vi "ShiftLeft.vi"(11 "Array":i32[](array[numeric])=[0, 3, 2, 1]) -> (3 "Array 2":i32[](array[numeric])=[0, 3, 2, 1], 5 "tiles moved?":bool)   [LabVIEW 2021]
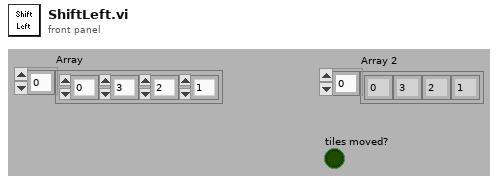
[diagram p1: front panel]
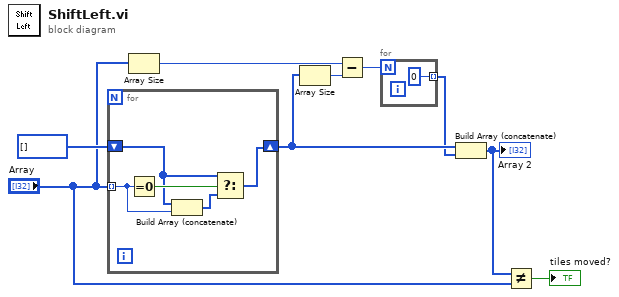
[diagram p0: block diagram]
diagram:
  n1 = for {
    tunnel: "Array" -> [w12] mode=indexing
    shift-right: [w13] -> w6
    shift-left: i32[] [] ("Array") -> [w10]
    n2 = Equal To 0?(x=w12) -> (x = 0?=w14:bool)
    n3 = Build Array (concatenate)(w10, w12) -> (w11:i32[])
    n4 = Select(t=w10, s=w14, f=w11) -> (s? t:f=w13:i32[])
  }
  n5 = Array Size(array="Array") -> (size(s)=w7:i32)
  n6 = Array Size(array=w6) -> (size(s)=w8:i32)
  n7 = Subtract(x=w7, y=w8) -> (x-y=w4:i32)
  n8 = for {
    N: w4 -> [_]
    tunnel: [0 ("Numeric")] -> w5 mode=indexing
  }
  n9 = Build Array (concatenate)(w6, w5) -> (w3:i32[])
  "Array 2" <- w3
  n10 = Not Equal?(x=w3, y="Array") -> (x != y?=→"tiles moved?":bool)
